vi "SubtractMeanFromPoints.vi"(8 "error in":errorcluster, 11 "x":T1) -> (0 "error out":errorcluster, 1 "var(x)":dbl format="%0.2f", 2 "mean(x)":dbl[](array[numeric]), 3 "x - mean(x)":dbl[][](array[numeric]))   [LabVIEW 2020, in "pointset_utils.lvlib" / "Affine Estimation.lvlib"]
uses:
  Affine Estimation.lvlib
  PointSet.ctl
  <vilib>/Analysis/baseanly.llb/Mean (DBL).vi
  <vilib>/ErrorRing/Error Ring.xnode
  <vilib>/Analysis/NI_AALBase.lvlib
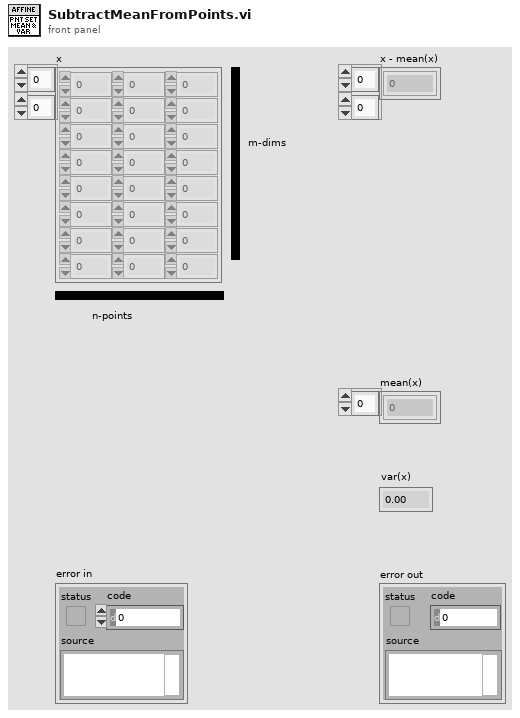
[diagram p1: front panel]
types:
  T1 = typedef "pointset_utils.lvlib/Affine Estimation.lvlib/PointSet.ctl" = dbl[][]
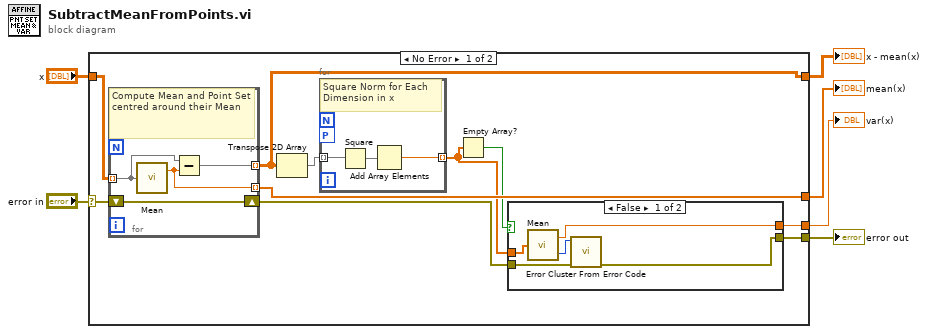
[diagram p0: block diagram]
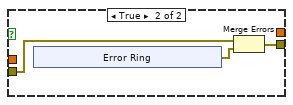
[diagram p2: hidden frame]
diagram:
  n1 = case shown="No Error" "error in" {
    selector: "error in" -> [w11 w37]
    tunnel: [w16 _] -> w6
    tunnel: "x" -> [w15 _]
    tunnel: [w13 _] -> w4
    tunnel: [w12 _] -> w3
    tunnel: [w9 w37] -> w1
    frame No Error {
      n2 = for {
        tunnel: w15 -> [w36] mode=indexing
        tunnel: [w35] -> w16 mode=indexing
        tunnel: [w34] -> w13 mode=indexing
        shift-right: [w33] -> w10
        shift-left: w11 -> [w33]
        # "Compute Mean and Point Set centred around their Mean"
        n3 = call-poly <vilib>:"Mean.vi"("X"=w36) -> ("mean"=w35:dbl)  [unwired: 1 out]
        n4 = Subtract(x=w36, y=w35) -> (x-y=w34:dbl[])
      }
      n5 = Transpose 2D Array(2D array=w13) -> (transposed array=w14:dbl[][])
      n6 = for {
        tunnel: w14 -> [w32] mode=indexing
        tunnel: [w30] -> w8 mode=indexing
        workers-P: _ -> [_]
        # "Square Norm for Each Dimension in x"
        n7 = Square(x=w32) -> (x^2=w31:dbl[])
        n8 = Add Array Elements(numeric array=w31) -> (sum=w30:dbl)
      }
      n9 = Empty Array?(array=w8) -> (empty?=w7:bool)
      n10 = case shown="False" w7 {
        tunnel: [w21 _] -> w12
        tunnel: w10 -> [w19 w24]
        tunnel: [w18 w23] -> w9
        tunnel: w8 -> [w17 _]
        frame False {
          n11 = call-poly <vilib>:"Mean.vi"("X"=w17) -> ("mean"=w21:dbl, "error"=w20:i32)
          n12 = call <vilib>:"Error Cluster From Error Code.vi"("error in (no error)"=w19, "error code (0)"=w20) -> ("error out"=w18:errorcluster)  [unwired: 7 in]
        }
        frame True {
          n13 = xnode "Error Ring"() -> ("error out"=w22:errorcluster)
          n14 = Merge Errors(w24, w22) -> (w23:errorcluster)
        }
      }
    }
    frame Error {
    }
  }
  "x - mean(x)" <- w4
  "mean(x)" <- w6
  "var(x)" <- w3
  "error out" <- w1
